vi "MainHost.vi"() -> ()   [LabVIEW 2021]
uses:
  <vilib>/LabVIEW Open Source Project/MQTT Client/Client class/Client.lvclass/Client.ctl
  <vilib>/LabVIEW Open Source Project/MQTT Connection/MQTT_Base/Base Class/MQTT_Base.lvclass/MQTT_Base.ctl
  <vilib>/LabVIEW Open Source Project/Connection/Connection.TCP/Connection.TCP.lvclass
  C:/Program Files (x86)/National Instruments/LabVIEW 2021/vi.lib/LabVIEW Open Source Project/Connection/Connection/Connection.lvclass
  <vilib>/LabVIEW Open Source Project/MQTT Client/Client class/Client.lvclass
  C:/Program Files (x86)/National Instruments/LabVIEW 2021/vi.lib/LabVIEW Open Source Project/MQTT Connection/MQTT_Base/Base Class/MQTT_Base.lvclass
  <vilib>/LabVIEW Open Source Project/MQTT Control Packets/Control Packets/PUBLISH/PUBLISH.lvclass
  <vilib>/LabVIEW Open Source Project/MQTT Connection/MQTT_Base/Base Class/MQTT_Base.lvclass
  <vilib>/LabVIEW Open Source Project/Connection/Connection.LocalQueue/Connection.LocalQueue.lvclass
  <vilib>/LabVIEW Open Source Project/Connection/Connection/Connection.lvclass
panel:
  out "Dados":string
  out "Unsuback":bool
  out "Suback":bool
  in  "Subscribe":bool
  in  "Connection":bool
  in  "Stop Client":bool
  out "last error":errorcluster
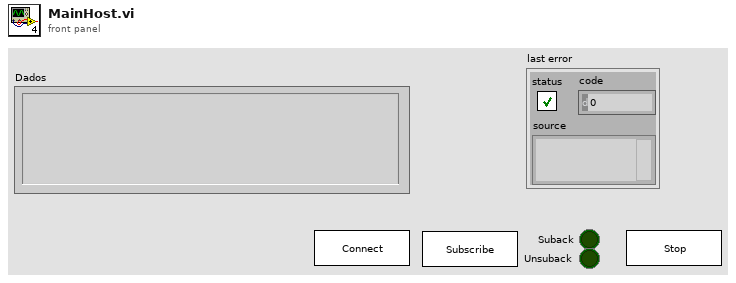
[diagram p1: front panel]
types:
  T1 = enum16{"open", "replace", "create", "open or create", "replace or create", "replace or create with confirmation"}
  T2 = typedef "MQTT Client.lvlib/Client.lvclass/Public Events -- cluster.ctl" = cluster{"Connection Status":refnum<user-event>, "Connected":refnum<user-event>, "Application Message":refnum<user-event>}
  T3 = typedef "MQTT Base.lvlib/MQTT_Base.lvclass/Public Events -- cluster.ctl" = cluster{"Stop Event":refnum<user-event>, "Error Event":refnum<user-event>, "Inbound Message":refnum<user-event>}
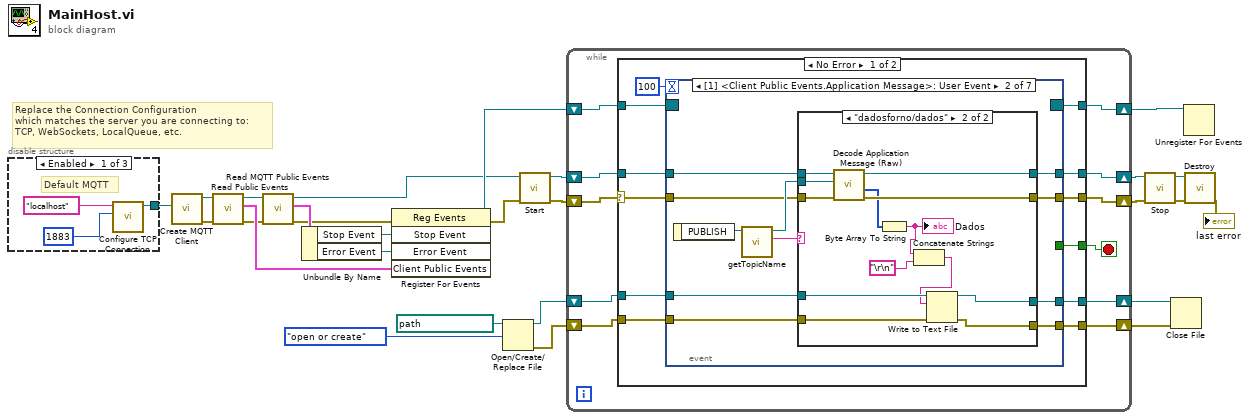
[diagram p0: block diagram]
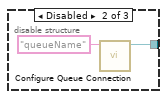
[diagram p2: hidden frame]
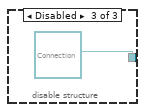
[diagram p3: hidden frame]
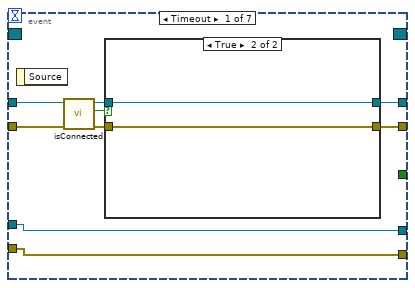
[diagram p4: hidden frame]
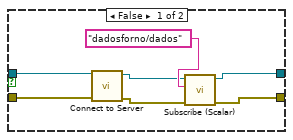
[diagram p5: hidden frame]
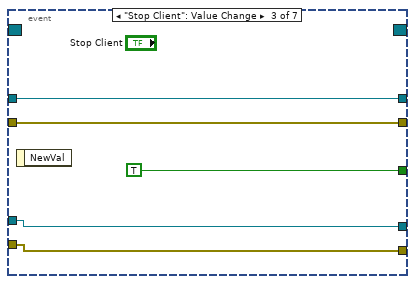
[diagram p7: hidden frame]
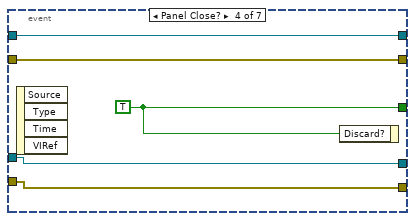
[diagram p8: hidden frame]
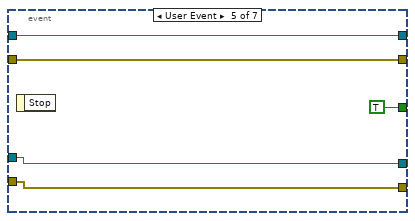
[diagram p9: hidden frame]
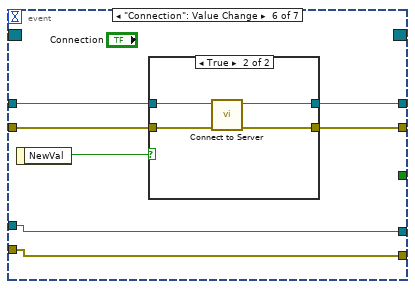
[diagram p10: hidden frame]
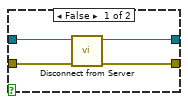
[diagram p11: hidden frame]
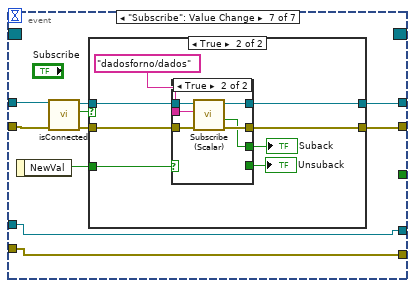
[diagram p12: hidden frame]
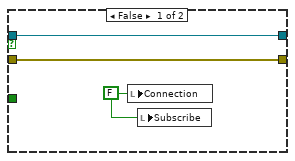
[diagram p13: hidden frame]
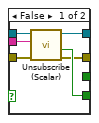
[diagram p14: hidden frame]
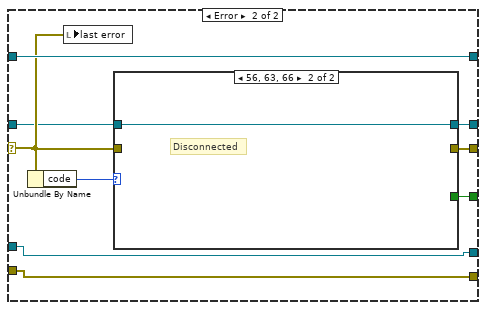
[diagram p15: hidden frame]
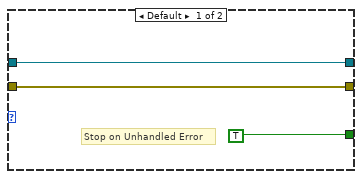
[diagram p16: hidden frame]
diagram:
  # "Replace the Connection Configuration\nwhich matches the server you are connecting to:\nTCP, WebSockets, LocalQueue, etc."
  n1 = disable-structure shown="Enabled" {
    disable-tunnel: [w29 w32 refnum<class "Connection.lvclass"> refnum ("Connection Configuration")] -> w27
    frame Enabled {
      # "Default MQTT"
      n2 = call <vilib>:"Configure TCP Connection.vi"("remote port (80)"=u16 1883, "address (localhost)"="localhost") -> ("Connection.TCP"=w29:refnum<class "Connection.TCP.lvclass">)  [unwired: 8 in, 1 out]
    }
    frame Disabled {
      n3 = call <vilib>:"Configure Queue Connection.vi"("Queue Name"="queueName") -> ("Connection.LocalQueue"=w32:refnum<class "Connection.LocalQueue.lvclass">)  [unwired: 9 in, 1 out]
    }
    frame Disabled {
    }
  }
  n4 = call <vilib>:"Create MQTT Client.vi"("Connection Configuration"=w27) -> ("error out"=w9:errorcluster, "Client out"=w7:refnum<class "Client.lvclass">)  [unwired: 9 in]
  n5 = call <vilib>:"Read Public Events.vi"("error in (no error)"=w9, "Client in"=w7) -> ("error out"=w10:errorcluster, "Client Public Events"=w12:T2, "Client out"=w8:refnum<class "Client.lvclass">)  [unwired: 7 in]
  n6 = call <vilib>:"Read MQTT Public Events.vi"("error in (no error)"=w10, "MQTT_Base in"=w8) -> ("error out"=w11:errorcluster, "MQTT Public Events"=w19:T3, "MQTT_Base out"=w14:refnum<class "Client.lvclass">)  [unwired: 7 in]
  n7 = Unbundle By Name(w19) -> ("Stop Event"=w17:refnum<user-event>, "Error Event"=w18:refnum<user-event>)
  n8 = register-events(error in=w11, w17, w18, w12) -> (reference out=w15:refnum<event-registration>, error out=w13:errorcluster)  [unwired: 1 in]
  n9 = Open/Create/Replace File(file path (use dialog)=path "D:/Videos em edição/x23 - Raspberry PZEM SPI quindim/Projeto/database.txt", operation (0:open)=T1."open or create") -> (refnum out=w4:refnum<file>, error out=w3:errorcluster)  [unwired: 4 in, 1 out]
  n10 = call <vilib>:"Start.vi"("error in (no error)"=w13, "MQTT_Base in"=w14) -> ("error out"=w25:errorcluster, "MQTT_Base out"=w24:refnum<class "Client.lvclass">)  [unwired: 7 in, 1 out]
  n11 = while {
    shift-right: [w43] -> w16
    shift-left: w15 -> [w44]
    shift-right: [w40] -> w21
    shift-left: w24 -> [w41]
    shift-right: [w42] -> w23
    shift-left: w25 -> [w38]
    shift-right: [w35] -> w2
    shift-left: w4 -> [w37]
    shift-right: [w34] -> w1
    shift-left: w3 -> [w36]
    stop <- w39 stop-if-true
    n12 = case shown="No Error" w38 {
      selector: w38 -> [w49 w171]
      tunnel: w44 -> [w56 w174]
      tunnel: [w55 w174] -> w43
      tunnel: [w54 w169] -> w42
      tunnel: w41 -> [w52 w170]
      tunnel: [w51 w173] -> w40
      tunnel: [w50 w168] -> w39
      tunnel: w37 -> [w48 w167]
      tunnel: w36 -> [w47 w166]
      tunnel: [w46 w167] -> w35
      tunnel: [w45 w166] -> w34
      frame No Error {
        n13 = event shown="[1] <Client Public Events.Application Message>: User Event" {
          selector: w56 -> [_ _ _ _ _ _ _]
          dyn-events: [_ _ _ _ _ _ _] -> w55
          timeout: 100 -> [_ _ _ _ _ _ _]
          tunnel: w49 -> [w61 w82 w106 w110 w117 w120 w140]
          tunnel: [w64 w79 w106 w110 w117 w121 w141] -> w54
          tunnel: [_ _ TRUE w112 TRUE _ _] -> w50
          tunnel: w52 -> [w63 w83 w107 w111 w115 w124 w139]
          tunnel: [w65 w81 w107 w111 w115 w122 w142] -> w51
          tunnel: w48 -> [w58 w78 w104 w109 w114 w119 w134]
          tunnel: w47 -> [w57 w77 w103 w108 w113 w118 w133]
          tunnel: [w58 w76 w104 w109 w114 w119 w134] -> w46
          tunnel: [w57 w75 w103 w108 w113 w118 w133] -> w45
          event Timeout {
            n14 = event-data() -> ()  [unwired: 1 in, 1 out]
            n15 = call <vilib>:"isConnected.vi"("error in (no error)"=w61, "Client in"=w63) -> ("error out"=w60:errorcluster, "connected"=w59:bool, "Client out"=w62:refnum<class "Client.lvclass">)  [unwired: 7 in]
            n16 = case shown="True" w59 {
              tunnel: [w67 w74] -> w65
              tunnel: [w66 w73] -> w64
              tunnel: w62 -> [w71 w74]
              tunnel: w60 -> [w72 w73]
              frame False {
                n17 = call <vilib>:"Connect to Server.vi"("error in (no error)"=w72, "Client in"=w71) -> ("error out"=w68:errorcluster, "Client out"=w69:refnum<class "Client.lvclass">)  [unwired: 6 in, 2 out]
                n18 = call <vilib>:"Subscribe (Scalar).vi"("error in (no error)"=w68, "Topic Filter"="dadosforno/dados" ("Topic Name (empty: Payload name)"), "Client in"=w69) -> ("error out"=w66:errorcluster, "Client out"=w67:refnum<class "Client.lvclass">)  [unwired: 6 in, 1 out]
              }
              frame True {
              }
            }
          }
          event User Event {
            n19 = event-data() -> ("PUBLISH"=w85:refnum<class "PUBLISH.lvclass">)  [unwired: 1 in]
            n20 = call <vilib>:"getTopicName.vi"("PUBLISH in"=w85) -> ("Topic"=w80:string, "PUBLISH out"=w84:refnum<class "PUBLISH.lvclass">)  [unwired: 8 in, 1 out]
            n21 = case shown="\"dadosforno/dados\"" w80 {
              tunnel: w84 -> [_ w100]
              tunnel: w83 -> [w89 w102]
              tunnel: w82 -> [w88 w101]
              tunnel: [w89 w99] -> w81
              tunnel: [w88 w98] -> w79
              tunnel: w78 -> [w87 w96]
              tunnel: w77 -> [w86 w95]
              tunnel: [w87 w94] -> w76
              tunnel: [w86 w93] -> w75
              frame Default {
              }
              frame "dadosforno/dados" {
                n22 = call <vilib>:"Decode Application Message (Raw).vi"("error in (no error)"=w101, "PUBLISH"=w100, "Client in"=w102) -> ("error out"=w98:errorcluster, "Payload"=w97:u8[], "Client out"=w99:refnum<class "Client.lvclass">)  [unwired: 5 in, 1 out]
                n23 = Byte Array To String(unsigned byte array=w97) -> (string=w92:string)
                "Dados" <- w92
                n24 = Concatenate Strings(w92, "\r\n") -> (w90:string)
                n25 = Write to Text File(file (use dialog)=w96, text=w90, error in=w95) -> (refnum out=w94:refnum<file>, error out=w93:errorcluster)  [unwired: 1 in, 1 out]
              }
            }
          }
          event "Stop Client": Value Change {
            n26 = event-data() -> ()  [unwired: 1 in, 1 out]
          }
          event Panel Close? {
            w112 = TRUE
            n27 = event-data() -> ()  [unwired: 1 in, 4 out]
            n28 = event-data("Discard?"=w112) -> ()  [unwired: 1 in, 1 out]
          }
          event User Event {
            n29 = event-data() -> ()  [unwired: 1 in, 1 out]
          }
          event "Connection": Value Change {
            n30 = event-data() -> ("NewVal"=w123:bool)  [unwired: 1 in]
            n31 = case shown="True" w123 {
              tunnel: w124 -> [w128 w132]
              tunnel: [w127 w129] -> w122
              tunnel: [w126 w130] -> w121
              tunnel: w120 -> [w125 w131]
              frame False {
                n32 = call <vilib>:"Disconnect from Server.vi"("error in (no error)"=w125, "Client in"=w128) -> ("error out"=w126:errorcluster, "Client out"=w127:refnum<class "Client.lvclass">)  [unwired: 7 in, 1 out]
              }
              frame True {
                n33 = call <vilib>:"Connect to Server.vi"("error in (no error)"=w131, "Client in"=w132) -> ("error out"=w130:errorcluster, "Client out"=w129:refnum<class "Client.lvclass">)  [unwired: 6 in, 2 out]
              }
            }
          }
          event "Subscribe": Value Change {
            n34 = event-data() -> ("NewVal"=w135:bool)  [unwired: 1 in]
            n35 = call <vilib>:"isConnected.vi"("error in (no error)"=w140, "Client in"=w139) -> ("error out"=w137:errorcluster, "connected"=w136:bool, "Client out"=w138:refnum<class "Client.lvclass">)  [unwired: 7 in]
            n36 = case shown="True" w136 {
              tunnel: [w145 w153] -> w142
              tunnel: [w144 w152] -> w141
              tunnel: w138 -> [w145 w151]
              tunnel: w137 -> [w144 w150]
              tunnel: w135 -> [_ w148]
              frame False {
                w143 = FALSE ("Connection")
                n37 = local write "Connection"(w143) -> ()
                n38 = local write "Subscribe"(w143) -> ()
              }
              frame True {
                n39 = case shown="True" w148 {
                  tunnel: [w154 w162] -> w153
                  tunnel: [w155 w161] -> w152
                  tunnel: w151 -> [w159 w165]
                  tunnel: w150 -> [w158 w164]
                  tunnel: "dadosforno/dados" ("Topic Name (empty: Payload name)") -> [w157 w163]
                  tunnel: [_ w160] -> w147
                  tunnel: [w156 _] -> w146
                  frame False {
                    n40 = call <vilib>:"Unsubscribe (Scalar).vi"("error in (no error)"=w158, "Topic Filter"=w157, "Client in"=w159) -> ("error out"=w155:errorcluster, "Ack"=w156:bool, "Client out"=w154:refnum<class "Client.lvclass">)  [unwired: 6 in]
                  }
                  frame True {
                    n41 = call <vilib>:"Subscribe (Scalar).vi"("error in (no error)"=w164, "Topic Filter"=w163, "Client in"=w165) -> ("error out"=w161:errorcluster, "Ack"=w160:bool, "Client out"=w162:refnum<class "Client.lvclass">)  [unwired: 6 in]
                  }
                }
                "Unsuback" <- w146
                "Suback" <- w147
              }
            }
          }
        }
      }
      frame Error {
        n42 = Unbundle By Name(w171) -> ("code"=w172:i32)
        n43 = local write "last error"(w171) -> ()
        n44 = case shown="56, 63, 66" w172 {
          tunnel: w170 -> [w177 w178]
          tunnel: [w177 w178] -> w173
          tunnel: w171 -> [w176 _]
          tunnel: [w176 _] -> w169
          tunnel: [TRUE _] -> w168
          frame Default {
            # "Stop on Unhandled Error"
          }
          frame 56, 63, 66 {
            # "Disconnected"
          }
        }
      }
    }
  }
  n45 = call <vilib>:"Stop.vi"("error in (no error)"=w23, "MQTT_Base in"=w21) -> ("error out"=w22:errorcluster, "MQTT_Base out"=w20:refnum<class "Client.lvclass">)  [unwired: 7 in, 1 out]
  n46 = Close File(refnum=w2, error in=w1) -> ()  [unwired: 2 out]
  n47 = Unregister For Events(event registration refnum=w16) -> ()  [unwired: 1 in, 1 out]
  n48 = call <vilib>:"Destroy.vi"("error in (no error)"=w22, "MQTT_Base in"=w20) -> ("error out"=→"last error":errorcluster)  [unwired: 8 in, 1 out]
